vi "set Data Write.vi"(6 "data":u32, 7 "data_pos":u16, 9 "data_length":u16, 10 "protocol_version":i32, 11 "port_num":i32) -> ()   [LabVIEW 2016, in "dxl_x86_c.lvlib"]
doc: "WINDECLSPEC void setDataWrite (int port_num, int protocol_version, uint16_t data_length, uint16_t data_pos, uint32_t data);"
uses:
  dxl_x86_c.lvlib
  dxl_x86_c.dll
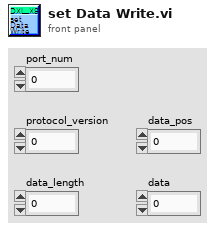
[diagram p1: front panel]
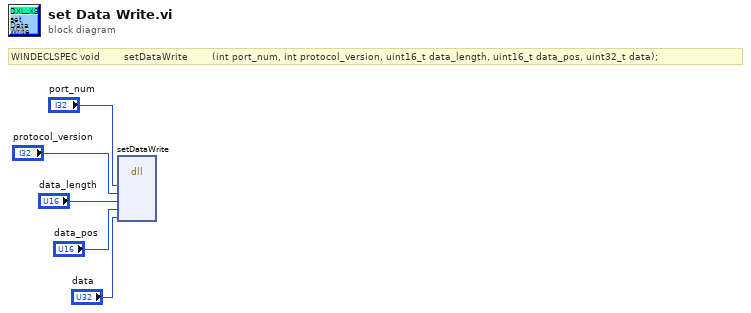
[diagram p0: block diagram]
diagram:
  # "WINDECLSPEC void        setDataWrite        (int port_num, int protocol_version, uint16_t data_length, uint16_t data_pos, uint32_t data);"
  n1 = dll-call lib="C:/Users/Platform/Desktop/DynamixelSDK/labview/dxl_x86_c.lvlib/dxl_x86_c.*" fn="setDataWrite"("port_num"="port_num", "protocol_version"="protocol_version", "data_length"="data_length", "data_pos"="data_pos", "data"="data") -> ()  [unwired: 9 in, 2 out]
